vi "LVFunction_Imop_BuildError.vi"(0 "code":i32, 5 "String to Prepend to source (\"\")":string, 7 "Adresse":i64, 9 "Activate error? (true)":bool=TRUE) -> (15 "error out":errorcluster)   [LabVIEW 2020]
doc: "Creates an error cluster, building the source string from the calling VIs call chain in a standard LabVIEW fashon. Builds source string as:\n\n\"<B>Calling VI</B> in <B>Calling VI's Caller</B>-><B>Calling VI's Caller's Caller</B>->etc...->etc...\"\n\nOptional 'String to Prepend to source (\"\")' string input is used to add extra descriptive info to the source string. This string, if present, will be enclosed in parenthesis and prepended to the source string."
panel:
  out "array w/ subset deleted 2":string[](array[string])
  out "array w/ subset deleted":string[](array[string])
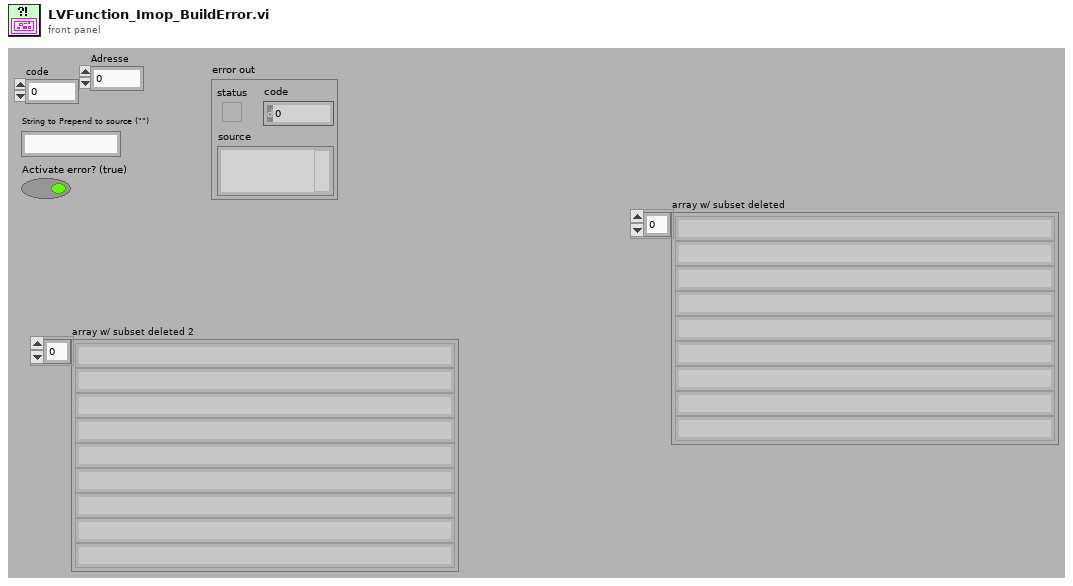
[diagram p1: front panel]
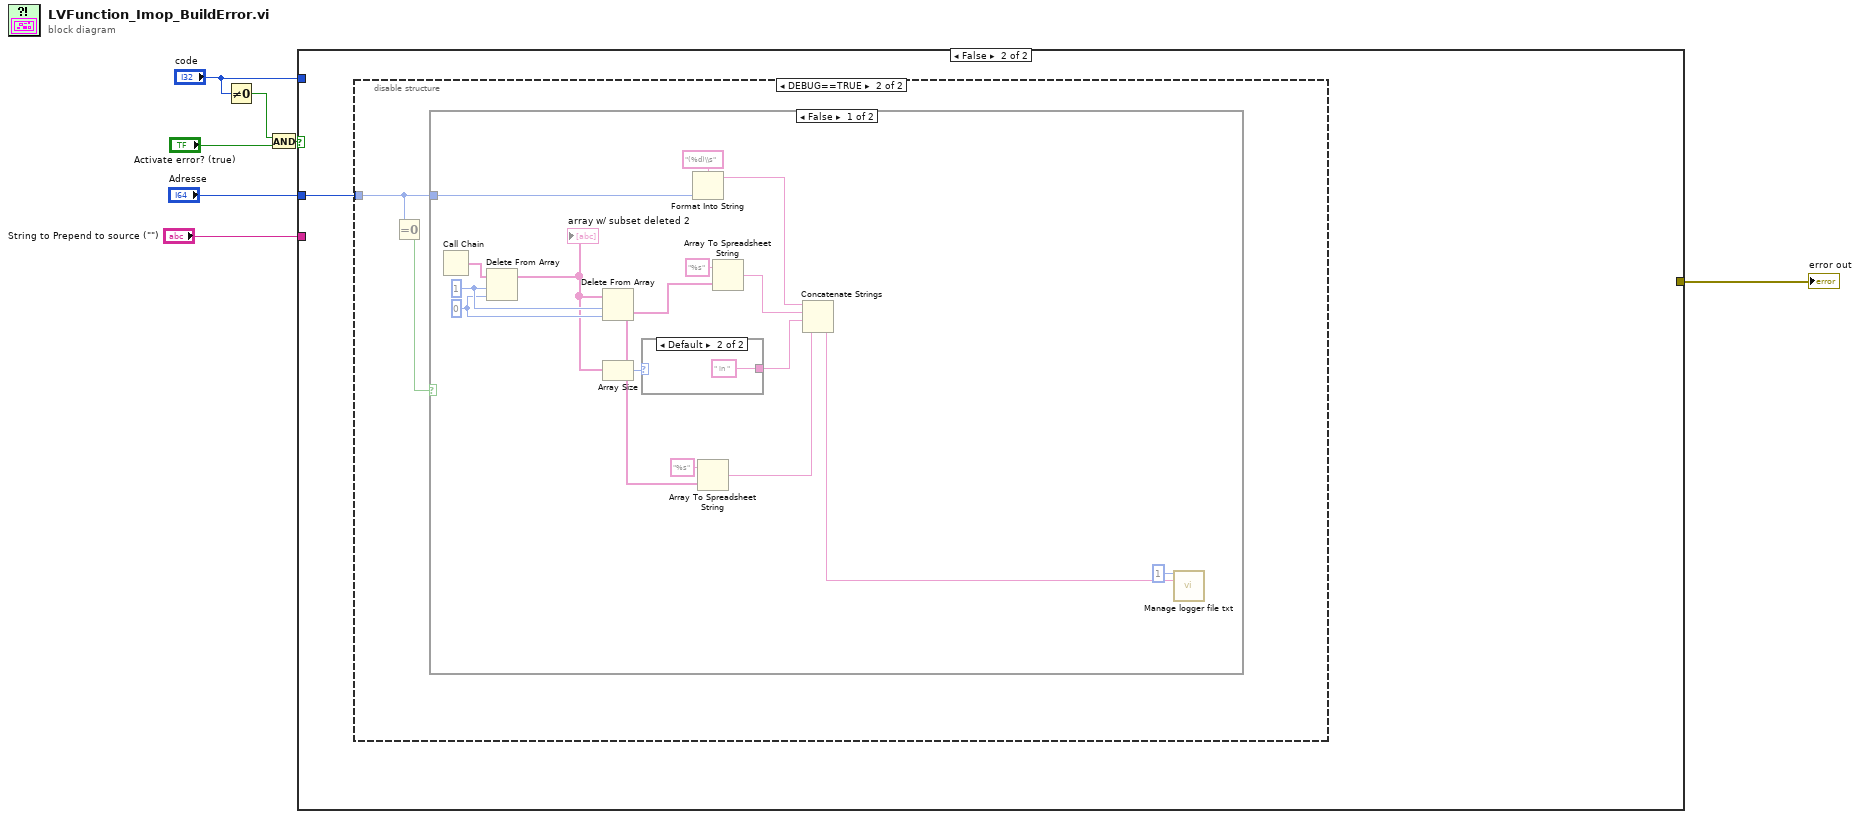
[diagram p0: block diagram]
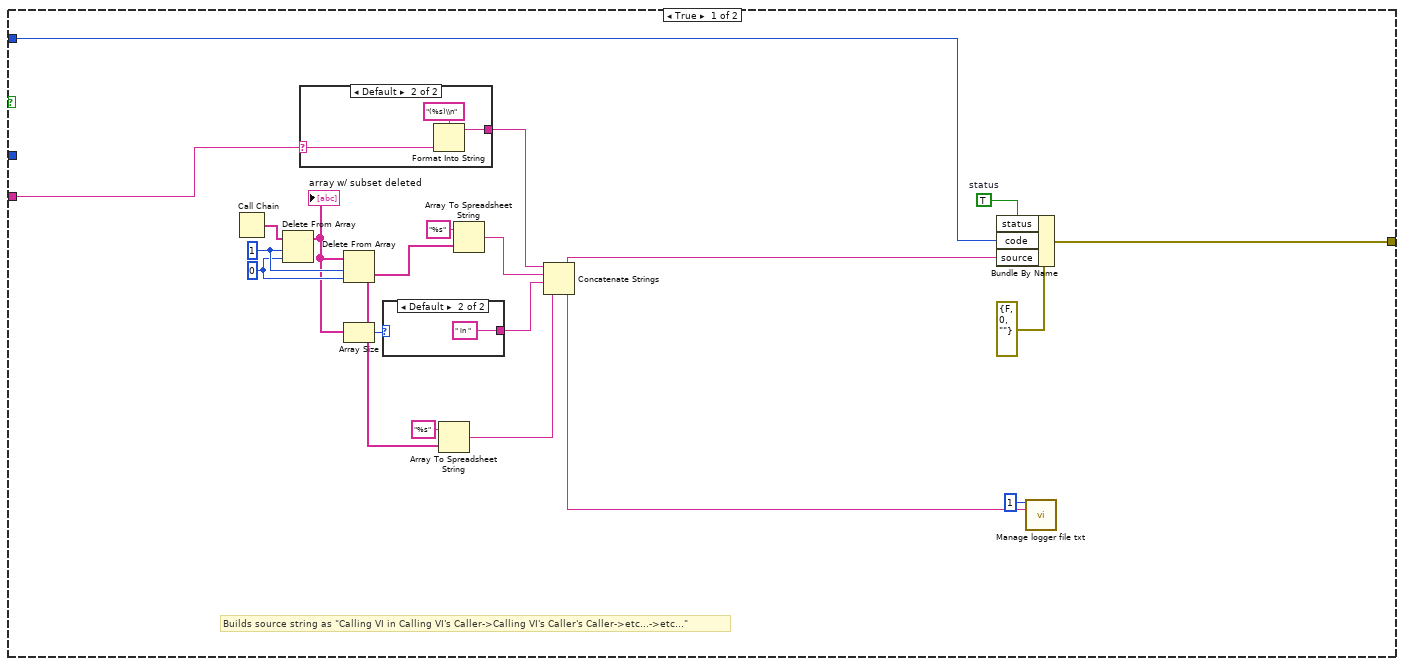
[diagram p2: hidden frame]
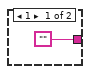
[diagram p3: hidden frame]
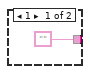
[diagram p6: hidden frame]
diagram:
  n1 = Not Equal To 0?(x="code") -> (x != 0?=w6:bool)
  n2 = And(x=w6, y="Activate error? (true)") -> (x .and. y?=w4:bool)
  n3 = case shown="False" w4 {
    tunnel: [w15 _] -> w7
    tunnel: "code" -> [w14 _]
    tunnel: "Adresse" -> [_ w34]
    tunnel: "String to Prepend to source (\"\")" -> [w8 _]
    frame True {
      w22 = 0 ("Index")
      w23 = 1 ("Length")
      w19 = TRUE  # status
      # "Builds source string as \"Calling VI in Calling VI's Caller->Calling VI's Caller's Caller->etc...->etc...\""
      n4 = Call Chain() -> (call chain=w27:string[])
      n5 = Delete From Array(array=w27, length=w23, index=w22) -> (array with subset deleted=w16:string[])  [unwired: 1 out]
      "array w/ subset deleted" <- w16
      n6 = case shown="Default" w8 {
        selector: w8 -> [w30 w33]
        tunnel: [w30 w31] -> w18
        frame "" {
        }
        frame Default {
          n7 = Format Into String(format string="(%s)\\n" ("Format String"), w33) -> (resulting string=w31:string)  [unwired: 2 in, 1 out]
        }
      }
      n8 = Delete From Array(array=w16, length=w23, index=w22) -> (deleted portion=w12:string[], array with subset deleted=w21:string[])
      n9 = Array Size(array=w16) -> (size(s)=w17:i32)
      n10 = case shown="Default" w17 {
        tunnel: ["" " in " ("Format String")] -> w26
        frame 1 {
        }
        frame Default {
        }
      }
      n11 = Array To Spreadsheet String(array=w21, 3:"%s" ("format string")) -> (spreadsheet string=w25:string)  [unwired: 1 in]
      n12 = Array To Spreadsheet String(array=w12, 3:"%s" ("format string")) -> (spreadsheet string=w11:string)  [unwired: 1 in]
      n13 = Concatenate Strings(w18, w11, w26, w25) -> (w9:string)
      n14 = Bundle By Name(cluster=errorcluster {"status"=FALSE, "code"=0, "source"=""} ("error out"), "status"=w19, "code"=w14, "source"=w9) -> (w15:errorcluster)
      n15 = call "Manage logger file txt.vi"("length"=1, "Message to add"=w9) -> ()  [unwired: 13 in, 1 out]
    }
    frame False {
      n16 = disable-structure shown="DEBUG==TRUE" {
        disable-tunnel: w34 -> [_ w36]
        frame condition #0 (active) {
        }
        frame condition #1 {
          n17 = Equal To 0?(x=w36) -> (x = 0?=w35:bool)
          n18 = case shown="False" w35 {
            tunnel: w36 -> [w37 _]
            frame False {
              w48 = 0 ("Index")
              w49 = 1 ("Length")
              n19 = Call Chain() -> (call chain=w53:string[])
              n20 = Delete From Array(array=w53, length=w49, index=w48) -> (array with subset deleted=w44:string[])  [unwired: 1 out]
              "array w/ subset deleted 2" <- w44
              n21 = Delete From Array(array=w44, length=w49, index=w48) -> (deleted portion=w42:string[], array with subset deleted=w47:string[])
              n22 = Array Size(array=w44) -> (size(s)=w45:i32)
              n23 = case shown="Default" w45 {
                tunnel: ["" " in " ("Format String")] -> w52
                frame 1 {
                }
                frame Default {
                }
              }
              n24 = Format Into String(format string="(%d)\\s" ("Format String"), w37) -> (resulting string=w46:string)  [unwired: 2 in, 1 out]
              n25 = Array To Spreadsheet String(array=w47, 3:"%s" ("format string")) -> (spreadsheet string=w51:string)  [unwired: 1 in]
              n26 = Array To Spreadsheet String(array=w42, 3:"%s" ("format string")) -> (spreadsheet string=w41:string)  [unwired: 1 in]
              n27 = Concatenate Strings(w46, w41, w52, w51) -> (w39:string)
              n28 = call "Manage logger file txt.vi"("length"=1, "Message to add"=w39) -> ()  [unwired: 13 in, 1 out]
            }
            frame True {
            }
          }
        }
      }
    }
  }
  "error out" <- w7
